vi "testFullCoverage.vi"() -> ()   [LabVIEW 2019, in "CodeCoverageTest.lvlib"]
uses:
  CodeCoverageTest.lvlib
  856f185b-f789-4ee0-abcd-cf80970f4a7f.vi
  CodeCoverageTestSupport/FakeUnit.vi
  Constraint/IsEqual/IsEqual.lvclass
  CodeCoverage/CodeCoverage.lvclass
  CodeCoverageTestSupport/CodeCoverageTestSupport.lvlib
panel:
  out "error out":errorcluster
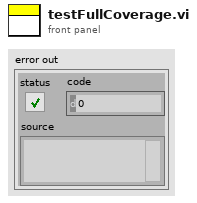
[diagram p1: front panel]
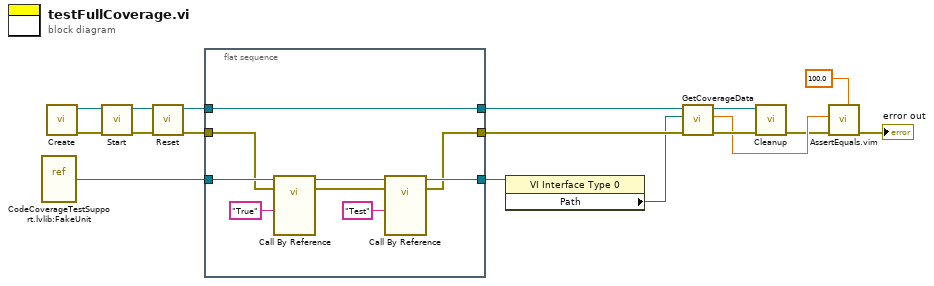
[diagram p0: block diagram]
diagram:
  n1 = vi-ref "CodeCoverageTestSupport.lvlib:FakeUnit.vi"() -> (w13:refnum<vi>)
  n2 = call "Create.vi"() -> ("error out"=w15:errorcluster, "CodeCoverage out"=w7:refnum<class "CodeCoverage.lvclass">)  [unwired: 10 in]
  n3 = call "Start.vi"("error in (no error)"=w15, "CodeCoverage in"=w7) -> ("error out"=w6:errorcluster, "CodeCoverage out"=w2:refnum<class "CodeCoverage.lvclass">)  [unwired: 8 in]
  n4 = call "Reset.vi"("error in (no error)"=w6, "CodeCoverage in"=w2) -> ("error out"=w3:errorcluster, "CodeCoverage out"=w1:refnum<class "CodeCoverage.lvclass">)  [unwired: 8 in]
  n5 = flat-sequence {
    tunnel: [w18] -> w16
    tunnel: w3 -> [w24]
    tunnel: [w20] -> w14
    tunnel: w13 -> [w26]
    tunnel: [w22] -> w12
    tunnel: w1 -> [w18]
    frame #0 {
      n6 = call-by-ref "?"(reference=w26, error in=w24, "Input"="True") -> (reference out=w23:refnum<vi>, error out=w21:errorcluster)  [unwired: 10 in, 1 out]
      n7 = call-by-ref "?"(reference=w23, error in=w21, "Input"="Test") -> (reference out=w22:refnum<vi>, error out=w20:errorcluster)  [unwired: 10 in, 1 out]
    }
  }
  n8 = property class="VI Interface Type 0"(reference=w12) -> ("Path"=w11:path)  [unwired: 1 in, 2 out]
  n9 = call "GetCoverageData.vi"("error in (no error)"=w14, "VI Path"=w11, "CodeCoverage in"=w16) -> ("error out"=w17:errorcluster, "Coverage Percentage"=w10:dbl, "CodeCoverage out"=w4:refnum<class "CodeCoverage.lvclass">)  [unwired: 6 in]
  n10 = call "Cleanup.vi"("error in (no error)"=w17, "CodeCoverage in"=w4) -> ("error out"=w5:errorcluster)  [unwired: 9 in]
  n11 = call "AssertEquals.vim"("Expected"=100.0, "error in (no error)"=w5, "Actual"=w10) -> ("error out"=→"error out":errorcluster)  [unwired: 8 in]
